vi "projeto.vi"() -> ()   [LabVIEW 2024]
uses:
  <vilib>/sound2/lvsound2.llb/Sampling Mode.ctl
  <vilib>/sound2/lvsound2.llb/Sound Data Format.ctl
  <vilib>/sound2/lvsound2.llb/Sound Output Set Volume (Single).vi
  <vilib>/sound2/lvsound2.llb/Sound Output Write (DBL Single).vi
panel:
  in  "volume":dbl(slide) scale=0.0..100.0 scale format="%1d"
  in  "E2":bool
  in  "D3":bool
  in  "E4":bool
  in  "G3":bool
  in  "B3":bool
  in  "A2":bool
  out "valor lido:":dbl
  in  "inserir valor\nmanualmente:":dbl
  out "valor da barra:":dbl
  in  "frequência":dbl(slide) scale=0.0..1000.0
  out "generated sound":waveform(dbl)(graph)
  in  "stop":bool
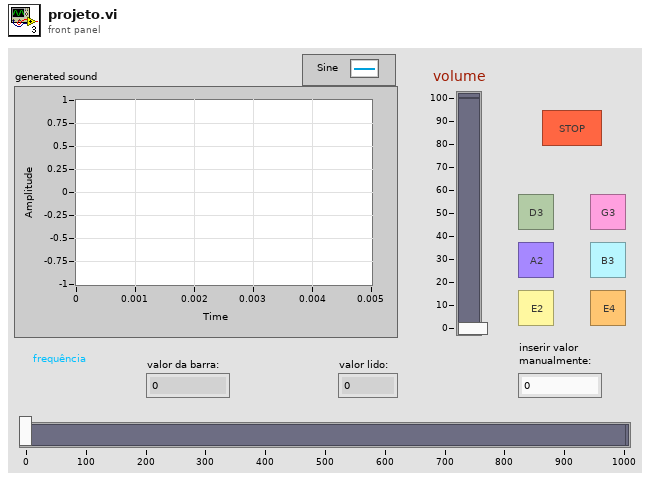
[diagram p1: front panel]
types:
  T1 = typedef "Sound Data Format.ctl" = cluster{"sample rate (S/s)":dbl, "number of channels":i32, "bits per sample":i32}
  T2 = typedef "Sampling Mode.ctl" = i32
  T3 = typedef "Sound Output Task ID.ctl" = u32
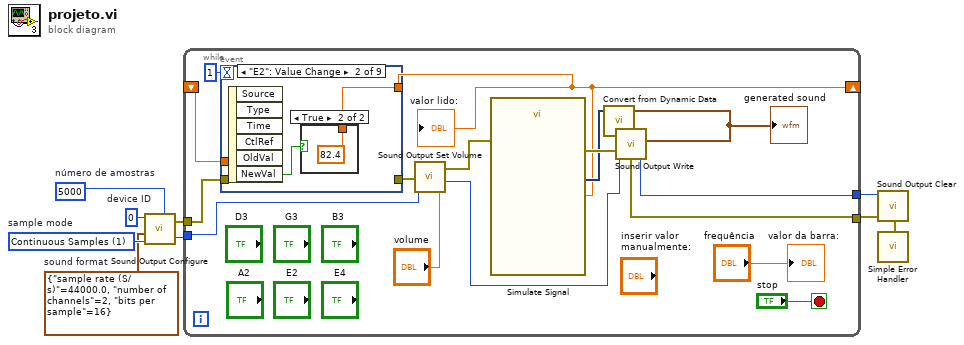
[diagram p0: block diagram]
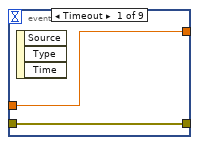
[diagram p2: hidden frame]
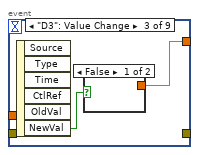
[diagram p4: hidden frame]
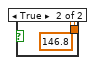
[diagram p5: hidden frame]
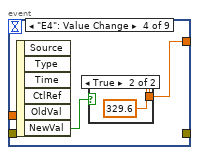
[diagram p6: hidden frame]
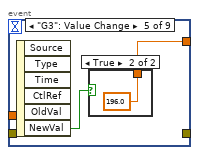
[diagram p8: hidden frame]
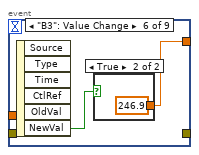
[diagram p10: hidden frame]
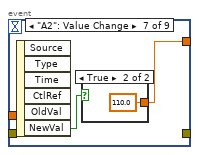
[diagram p12: hidden frame]
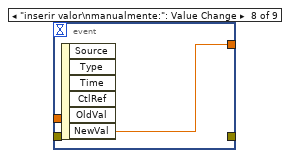
[diagram p14: hidden frame]
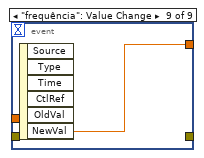
[diagram p15: hidden frame]
diagram:
  w6 = 0  # device ID
  w8 = 5000  # número de amostras
  w7 = T1 {"sample rate (S/s)"=44000.0, "number of channels"=2, "bits per sample"=16}  # sound format
  w9 = T2 1 items=["Finite Samples", "Continuous Samples"]  # sample mode
  n1 = call <vilib>:"Sound Output Configure.vi"("number of samples/ch"=w8, "sample mode"=w9, "sound format"=w7, "device ID"=w6) -> ("error out"=w4:errorcluster, "task ID"=w5:T3)  [unwired: 6 in]
  n2 = while {
    tunnel: w5 -> [w10]
    tunnel: w4 -> [w15]
    tunnel: [w22] -> w2
    tunnel: [w21] -> w3
    shift-right: [w11] -> _
    shift-left: _ -> [w13]
    stop <- "stop" stop-if-true
    n3 = event shown="[1] \"E2\": Value Change" {
      selector: _ -> [_ _ _ _ _ _ _ _ _]
      dyn-events: _ -> [_ _ _ _ _ _ _ _ _]
      timeout: 1 -> [_ _ _ _ _ _ _ _ _]
      tunnel: [w27 _ _ _ _ _ _ _ _] -> w16
      tunnel: w15 -> [w27 _ _ _ _ _ _ _ _]
      tunnel: [w26 w28 w31 w34 w37 w40 w43 w46 w47] -> w11
      tunnel: w13 -> [w26 _ _ _ _ _ _ _ _]
      event Timeout {
        n4 = event-data() -> ()  [unwired: 1 in, 3 out]
      }
      event "E2": Value Change {
        n5 = event-data() -> ("NewVal"=w29:bool)  [unwired: 1 in, 5 out]
        n6 = case shown="True" w29 {
          tunnel: [_ 82.4] -> w28
          frame False {
          }
          frame True {
          }
        }
      }
      event "D3": Value Change {
        n7 = event-data() -> ("NewVal"=w32:bool)  [unwired: 1 in, 5 out]
        n8 = case shown="False" w32 {
          tunnel: [_ 146.8] -> w31
          frame False {
          }
          frame True {
          }
        }
      }
      event "E4": Value Change {
        n9 = event-data() -> ("NewVal"=w35:bool)  [unwired: 1 in, 5 out]
        n10 = case shown="True" w35 {
          tunnel: [_ 329.6] -> w34
          frame False {
          }
          frame True {
          }
        }
      }
      event "G3": Value Change {
        n11 = event-data() -> ("NewVal"=w38:bool)  [unwired: 1 in, 5 out]
        n12 = case shown="True" w38 {
          tunnel: [_ 196.0] -> w37
          frame False {
          }
          frame True {
          }
        }
      }
      event "B3": Value Change {
        n13 = event-data() -> ("NewVal"=w41:bool)  [unwired: 1 in, 5 out]
        n14 = case shown="True" w41 {
          tunnel: [_ 246.9] -> w40
          frame False {
          }
          frame True {
          }
        }
      }
      event "A2": Value Change {
        n15 = event-data() -> ("NewVal"=w44:bool)  [unwired: 1 in, 5 out]
        n16 = case shown="True" w44 {
          tunnel: [_ 110.0] -> w43
          frame False {
          }
          frame True {
          }
        }
      }
      event "inserir valor\nmanualmente:": Value Change {
        n17 = event-data() -> ("NewVal"=w46:dbl)  [unwired: 1 in, 5 out]
      }
      event "frequência": Value Change {
        n18 = event-data() -> ("NewVal"=w47:dbl)  [unwired: 1 in, 5 out]
      }
    }
    "valor lido:" <- w11
    n19 = call-poly <vilib>:"Sound Output Set Volume.vi"("error in (no error)"=w16, "volume"="volume", "task ID"=w10) -> ("error out"=w25:errorcluster, "task ID out"=w23:T3)  [unwired: 7 in]
    n20 = call "Simulate Signal"("Frequency"=w11, "error in (no error)"=w25) -> ("Sine"=w18:dynamicdata, "error out"=w24:errorcluster)  [unwired: 12 in]
    n21 = call "Convert from Dynamic Data"("Dynamic Data Type"=w18) -> ("Waveform"=w19:waveform(dbl))  [unwired: 3 in]
    "generated sound" <- w19
    n22 = call-poly <vilib>:"Sound Output Write.vi"("error in (no error)"=w24, "data"=w19, "task ID"=w23) -> ("error out"=w22:errorcluster, "task ID out"=w21:T3)  [unwired: 7 in]
    "valor da barra:" <- "frequência"
  }
  n23 = call <vilib>:"Sound Output Clear.vi"("error in (no error)"=w2, "task ID"=w3) -> ("error out"=w1:errorcluster)  [unwired: 9 in]
  n24 = call <vilib>:"Simple Error Handler.vi"("error in (no error)"=w1) -> ()  [unwired: 4 in, 5 out]
